vi "Safety_Check.vi"(1 "Adam Loop Count":i32, 2 "Ch Names":string[](array[string]), 3 "Values":dbl[](array[numeric]) format="%.2f") -> (0 "Scan comment":string)   [LabVIEW 2013]
uses:
  ADAM Client/Sub VIs/ADAM Controls/Update_scan_value.ctl
  Anemometry/Anemometry Sub Vis/Globals/Gas_management_global.vi
  ADAM_Global.vi
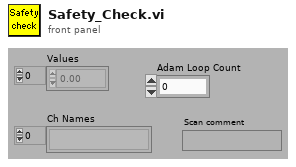
[diagram p1: front panel]
types:
  T1 = cluster{"Channel name":string, "Set value of A to":dbl, "Set value of B to":dbl, "Set value of C to":dbl, "Set value of D to":dbl}
  T2 = typedef "Update_scan_value.ctl" = cluster{"Channel Name":string, "New Value":dbl}
  T3 = enum16{"Append to Global", "Read Global then Clear"}
  T4 = enum16{"On", "Off", "Always On", "Always Off", "Delete"}
  T5 = typedef "LVDateTimeRec.ctl" = cluster{"fractional second":dbl, "second":i32, "minute":i32, "hour":i32, "day of month":i32, "month":i32, "year":i32, "day of week":i32, "day of year":i32, "DST":i32}
  T6 = cluster{"Channel name":string, "Set value of A to":dbl, "Set value of B to":dbl, "Set value of C to":dbl, "Set value of D to":dbl}[]
  T7 = typedef "Ch_description_ADAM.ctl" = cluster{"Ch Name":string, "Type":T8, "Function":T9, "Ch State":T10, "Calibration type":T11, "A":dbl, "B":dbl, "C":dbl, "D":dbl, "Comments":string, "Address":T12, "String":string, "Duty":u16}
  T8 = typedef "Module_type_ADAM.ctl" = string
  T9 = typedef "Function_ADAM.ctl" = enum16{"Analogue Input", "Digital Input", "Event counter", "Event rate", "Analogue Output", "Digital Output", "Relay Output"}
  T10 = typedef "Channel_State.ctl" = enum16{"On", "Off", "Always On", "Always Off"}
  T11 = typedef "Calib_type_ADAM.ctl" = enum16{"Raw", "Bx + A", "Cx^2 + Bx + A", "Dx^3 + Cx^2 + Bx + A", "In Band", "Hi-Tec Q", "Hi-Tec M_dot", "Text"}
  T12 = typedef "Address.ctl" = cluster{"Main":i32, "Ch.":i32, "Sub":i32, "Port Name":string}
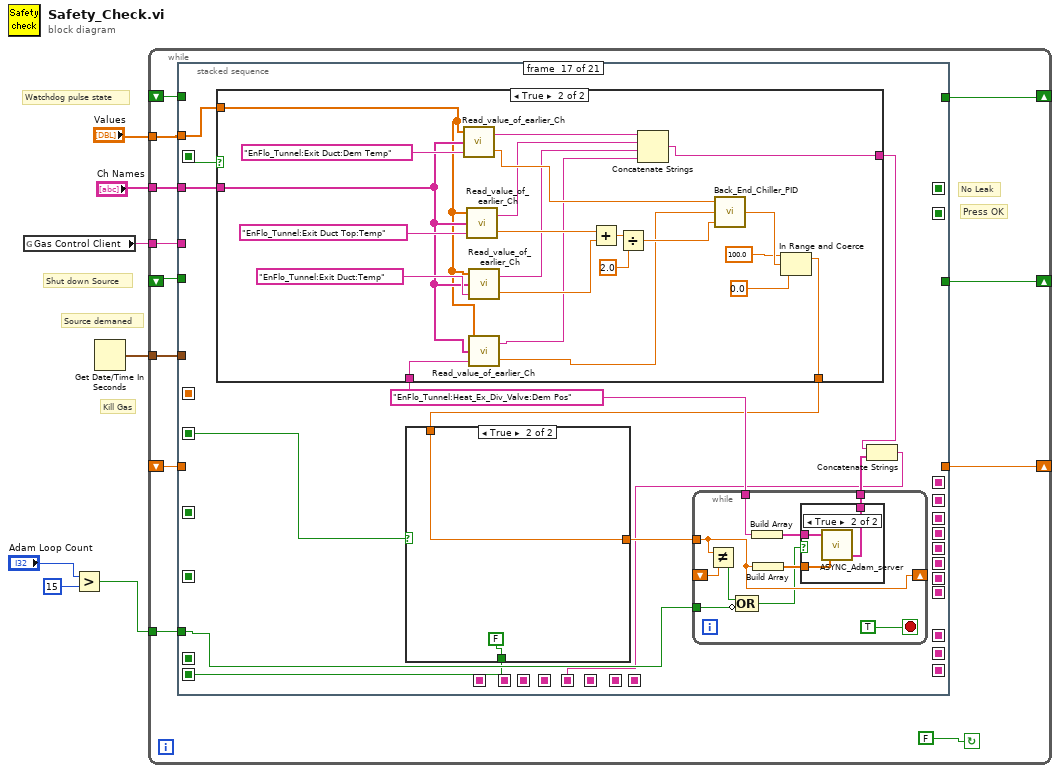
[diagram p0: block diagram]
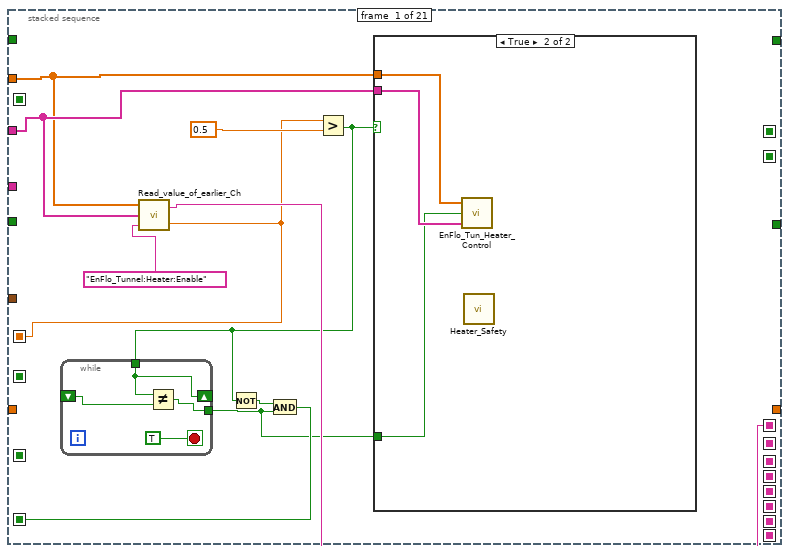
[diagram p2: hidden frame]
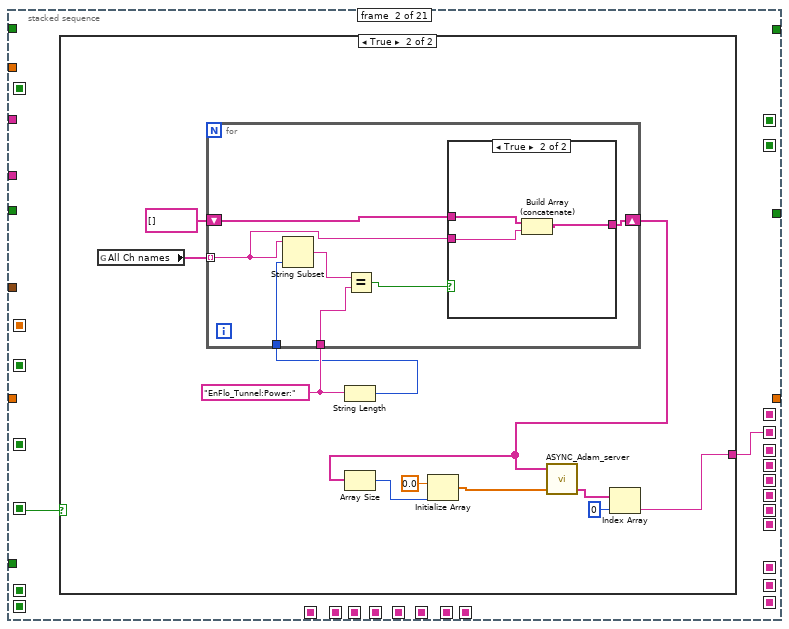
[diagram p4: hidden frame]
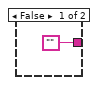
[diagram p5: hidden frame]
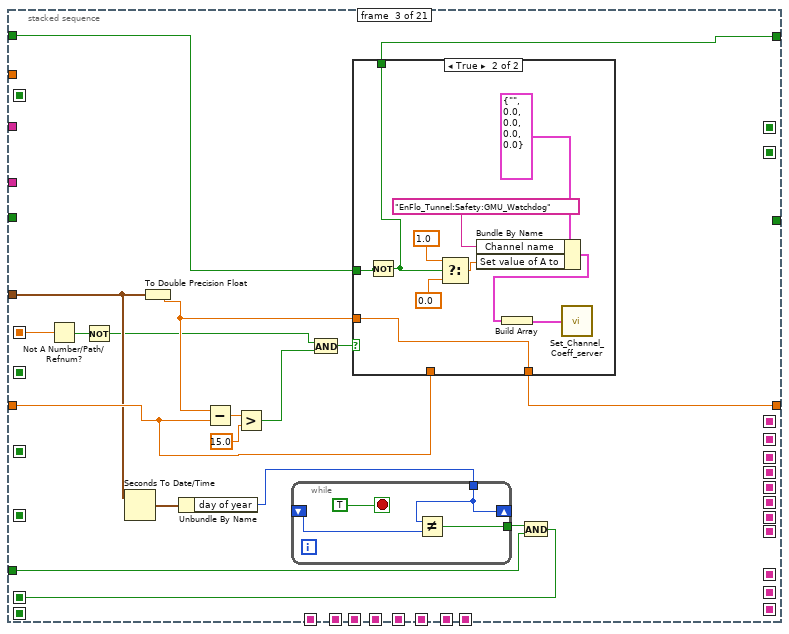
[diagram p7: hidden frame]
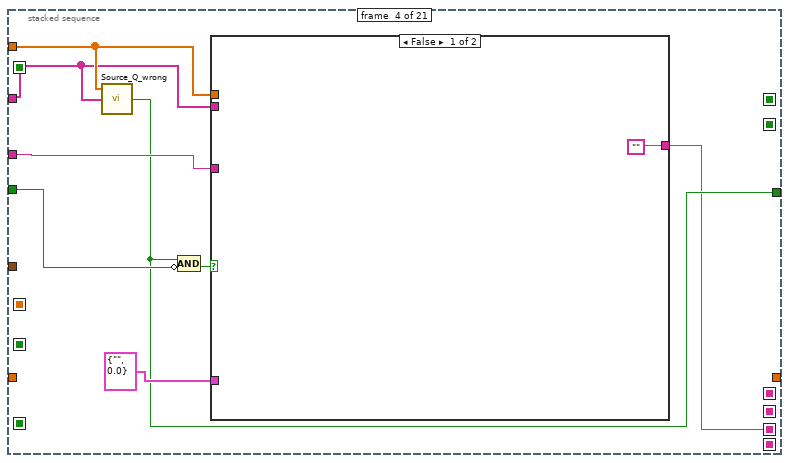
[diagram p9: hidden frame]
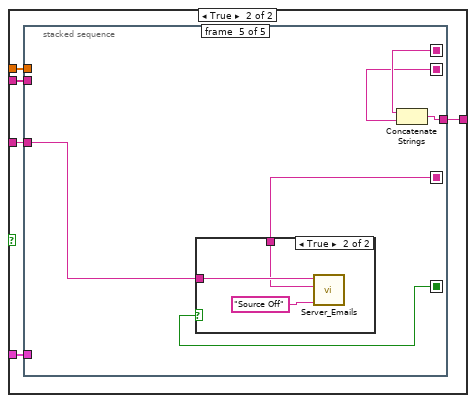
[diagram p10: hidden frame]
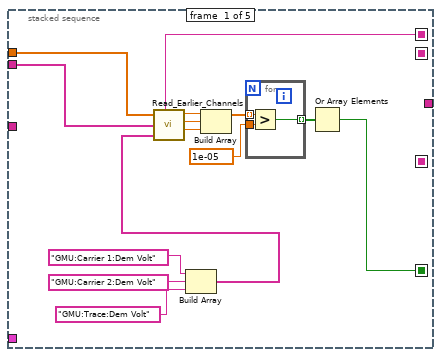
[diagram p11: hidden frame]
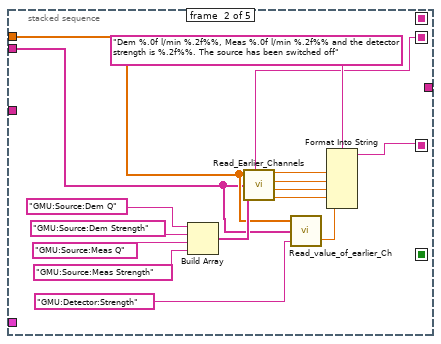
[diagram p12: hidden frame]
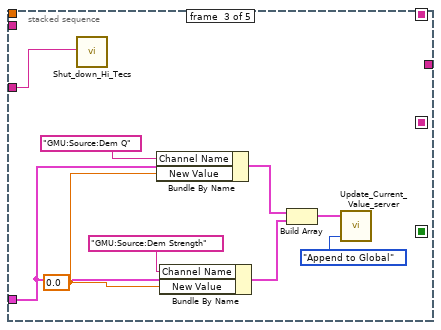
[diagram p13: hidden frame]
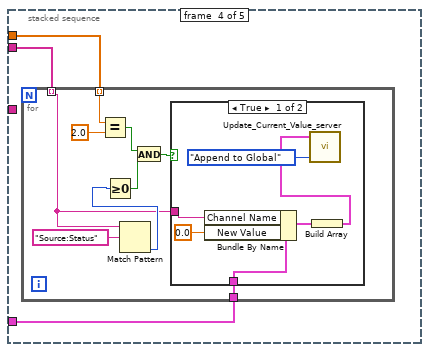
[diagram p14: hidden frame]
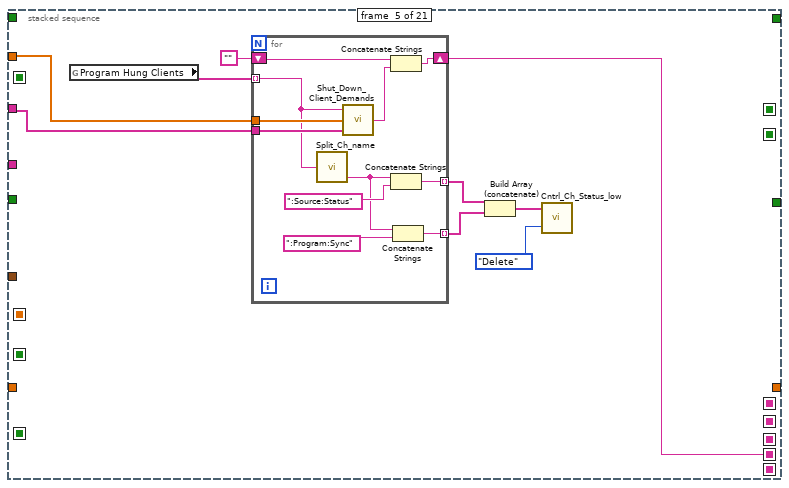
[diagram p17: hidden frame]
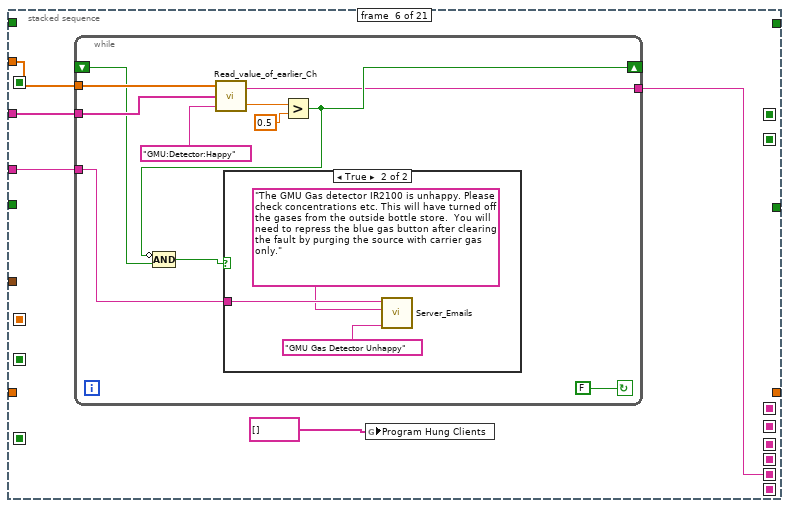
[diagram p18: hidden frame]
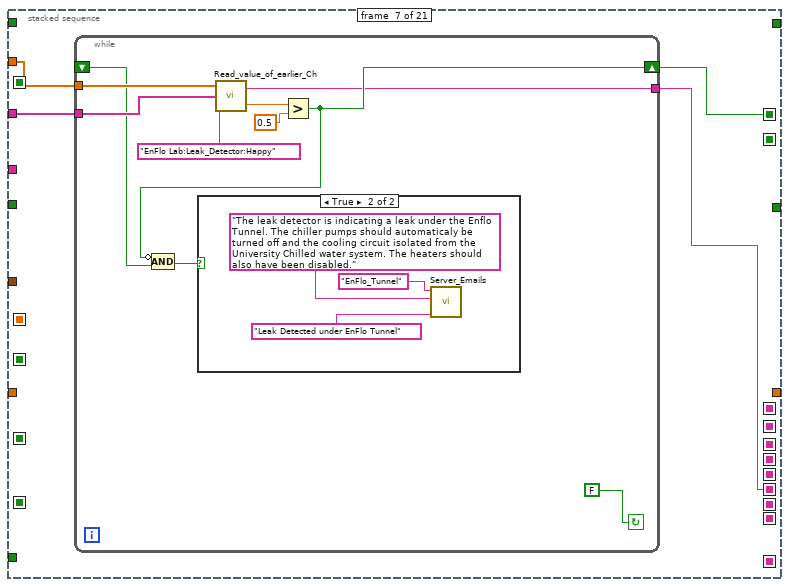
[diagram p20: hidden frame]
diagram:
  # "Shut down Source"
  # "Source demaned"
  # "Watchdog pulse state"
  # "Kill Gas"
  n1 = global read "Gas_management_global.vi" "Gas Control Client"() -> (w5:string)
  n2 = Greater?(x="Adam Loop Count", y=15) -> (0:w2:bool)
  n3 = Get Date/Time In Seconds() -> (seconds since 1Jan1904=w1:timestamp)
  n4 = while {
    shift-left: _ -> [w14]
    shift-right: [w13] -> _
    shift-left: _ -> [w16]
    shift-right: [w15] -> _
    tunnel: w5 -> [w18]
    tunnel: "Ch Names" -> [w19]
    tunnel: "Values" -> [w17]
    shift-right: [w11] -> _
    shift-left: _ -> [w10]
    tunnel: w2 -> [w9]
    tunnel: w1 -> [w8]
    stop <- FALSE continue-if-true
    # "Press OK"
    # "No Leak"
    n5 = stacked-sequence {
      seq-local: [_ _ _ _ _ _ w219 _ _ _ _ _ _ _ _ _ _ _ _ _ _] -> [_ _ _ _ _ _ _ _ _ _ _ _ _ w453 _ _ _ _ _ _ _]
      seq-local: [w22 _ _ _ _ _ _ _ _ _ _ _ _ _ _ _ _ _ _ _ _] -> [_ w38 _ _ _ _ _ _ _ _ _ _ _ _ _ _ _ _ _ _ _]
      seq-local: [_ _ w68 _ _ _ _ _ _ _ _ _ _ _ _ _ _ _ _ _ _] -> [_ _ _ _ _ _ _ _ _ _ _ _ _ _ _ _ _ _ _ _ _]
      seq-local: [_ _ _ _ _ _ _ _ _ _ _ _ _ _ _ w514 _ _ _ _ _] -> [_ _ _ _ _ _ _ _ _ _ _ _ _ _ _ _ w527 _ _ _ _]
      seq-local: [_ _ _ _ _ _ _ _ _ _ _ _ _ _ _ _ w522 _ _ _ _] -> [_ _ _ _ _ _ _ _ _ _ _ _ _ _ _ _ _ _ _ w648 _]
      seq-local: [w25 _ _ _ _ _ _ _ _ _ _ _ _ _ _ _ _ _ _ _ _] -> [_ _ _ _ _ _ _ _ _ _ _ _ _ _ _ _ _ _ _ _ w685]
      seq-local: [_ w37 _ _ _ _ _ _ _ _ _ _ _ _ _ _ _ _ _ _ _] -> [_ _ _ _ _ _ _ _ _ _ _ _ _ _ _ _ _ _ _ _ w684]
      seq-local: [_ _ _ w96 _ _ _ _ _ _ _ _ _ _ _ _ _ _ _ _ _] -> [_ _ _ _ _ _ _ _ _ _ _ _ _ _ _ _ _ _ _ _ w683]
      seq-local: [_ _ _ _ w179 _ _ _ _ _ _ _ _ _ _ _ _ _ _ _ _] -> [_ _ _ _ _ _ _ _ _ _ _ _ _ _ _ _ _ _ _ _ w682]
      seq-local: [_ _ _ _ _ w199 _ _ _ _ _ _ _ _ _ _ _ _ _ _ _] -> [_ _ _ _ _ _ _ _ _ _ _ _ _ _ _ _ _ _ _ _ w681]
      seq-local: [_ _ _ _ _ _ w218 _ _ _ _ _ _ _ _ _ _ _ _ _ _] -> [_ _ _ _ _ _ _ _ _ _ _ _ _ _ _ _ _ _ _ _ w680]
      seq-local: [_ _ _ _ _ _ _ _ _ w330 _ _ _ _ _ _ _ _ _ _ _] -> [_ _ _ _ _ _ _ _ _ _ _ _ _ _ _ _ _ _ _ _ w679]
      seq-local: [_ _ _ _ _ _ _ _ _ _ w362 _ _ _ _ _ _ _ _ _ _] -> [_ _ _ _ _ _ _ _ _ _ _ _ _ _ _ _ _ _ _ _ w670]
      seq-local: [_ _ _ _ _ _ _ _ _ _ _ _ w430 _ _ _ _ _ _ _ _] -> [_ _ _ _ _ _ _ _ _ _ _ _ _ _ _ _ _ _ _ _ w669]
      seq-local: [_ _ _ _ _ _ _ _ _ _ _ _ _ w454 _ _ _ _ _ _ _] -> [_ _ _ _ _ _ _ _ _ _ _ _ _ _ _ _ _ _ _ _ w672]
      seq-local: [_ _ _ _ _ _ _ _ _ _ _ _ _ _ w481 _ _ _ _ _ _] -> [_ _ _ _ _ _ _ _ _ _ _ _ _ _ _ _ _ _ _ _ w673]
      seq-local: [_ _ _ _ _ _ _ _ _ _ _ _ _ _ _ w505 _ _ _ _ _] -> [_ _ _ _ _ _ _ _ _ _ _ _ _ _ _ _ _ _ _ _ w674]
      seq-local: [_ _ _ _ _ _ _ _ _ _ _ _ _ _ _ _ w519 _ _ _ _] -> [_ _ _ _ _ _ _ _ _ _ _ _ _ _ _ _ _ _ _ _ w675]
      seq-local: [_ _ _ _ _ _ _ _ _ _ _ _ _ _ _ _ _ w581 _ _ _] -> [_ _ _ _ _ _ _ _ _ _ _ _ _ _ _ _ _ _ _ _ w676]
      seq-local: [_ _ _ _ _ _ _ _ _ _ _ _ _ _ _ _ _ _ w610 _ _] -> [_ _ _ _ _ _ _ _ _ _ _ _ _ _ _ _ _ _ _ _ w677]
      seq-local: [_ _ _ _ _ _ _ _ _ _ _ _ _ _ _ _ _ _ _ w646 _] -> [_ _ _ _ _ _ _ _ _ _ _ _ _ _ _ _ _ _ _ _ w678]
      seq-local: [w24 _ _ _ _ _ _ _ _ _ _ _ _ _ _ _ _ _ _ _ _] -> [_ _ w66 _ _ _ _ _ _ _ _ _ _ _ _ _ _ _ _ _ _]
      seq-local: [_ _ _ _ _ _ _ _ _ _ _ _ _ _ _ w504 _ _ _ _ _] -> [_ _ _ _ _ _ _ _ _ _ _ _ _ _ _ _ w518 _ _ _ _]
      seq-local: [_ _ _ _ _ _ _ w237 _ _ _ _ _ _ _ _ _ _ _ _ _] -> [_ _ _ _ _ _ _ _ _ _ _ _ _ w452 _ _ _ _ _ _ _]
      seq-local: [_ _ _ _ _ _ _ w236 _ _ _ _ _ _ _ _ _ _ _ _ _] -> [_ _ _ _ _ _ _ _ _ _ _ _ _ _ _ _ _ _ _ _ w668]
      seq-local: [_ _ _ _ _ _ _ w235 _ _ _ _ _ _ _ _ _ _ _ _ _] -> [_ _ _ _ _ _ _ _ w267 _ _ _ _ _ _ _ _ _ _ _ _]
      seq-local: [_ _ _ _ _ _ _ _ w264 _ _ _ _ _ _ _ _ _ _ _ _] -> [_ _ _ _ _ _ _ _ _ _ _ _ _ _ _ _ _ _ _ _ _]
      seq-local: [_ _ _ _ _ _ _ _ _ _ _ w384 _ _ _ _ _ _ _ _ _] -> [_ _ _ _ _ _ _ _ _ _ _ _ _ _ _ _ _ _ _ _ w667]
      tunnel: w19 -> [w27 _ _ w98 w186 w201 w220 w238 w265 w331 w363 w385 w432 w455 w487 w510 w528 w586 w613 _ _]
      tunnel: w18 -> [_ _ _ w103 _ w200 _ _ _ _ _ _ _ _ _ _ _ _ _ _ _]
      tunnel: w17 -> [w26 _ _ w99 w182 w202 w221 w239 w266 w332 w364 w386 w433 w456 w488 w511 w529 w587 w614 _ _]
      tunnel: w16 -> [_ _ w79 _ _ _ _ _ _ _ _ _ _ _ _ _ _ _ _ _ _]
      tunnel: [_ _ w78 _ _ _ _ _ _ _ _ _ _ _ _ _ _ _ _ _ _] -> w15
      tunnel: w14 -> [_ _ _ w102 _ _ _ _ _ _ _ _ _ _ _ _ _ _ _ _ _]
      tunnel: [_ _ _ w97 _ _ _ _ _ _ _ _ _ _ _ _ _ _ _ _ _] -> w13
      tunnel: [_ _ w77 _ _ _ _ _ _ _ _ _ _ _ _ _ _ _ _ _ _] -> w11
      tunnel: w10 -> [_ _ w73 _ _ _ _ _ _ _ _ _ _ _ _ _ _ _ _ _ _]
      tunnel: w9 -> [_ _ w69 _ _ _ _ _ _ _ _ w382 w431 _ _ _ w523 w582 _ w647 _]
      tunnel: w8 -> [_ _ w67 _ _ _ _ _ _ _ _ w383 _ _ _ _ _ _ _ _ _]
      frame #0 {
        n6 = call "Read_value_of_earlier_Ch.vi"("Desired Ch to Read"="EnFlo_Tunnel:Heater:Enable", "Ch names"=w27, "Present scan array"=w26) -> ("Value"=w24:dbl, "Scan comment"=w25:string)  [unwired: 1 in]
        n7 = Greater?(x=w24, y=0.5) -> (0:w23:bool)
        n8 = while {
          shift-right: [w33] -> _
          shift-left: _ -> [w32]
          tunnel: w23 -> [w33]
          tunnel: [w30] -> w20
          stop <- TRUE stop-if-true
          n9 = Not Equal?(x=w33, y=w32) -> (x != y?=w30:bool)
        }
        n10 = Not(x=w23) -> (.not. x?=w21:bool)
        n11 = And(x=w21, y=w20) -> (x .and. y?=w22:bool)
        n12 = case shown="True" w23 {
          tunnel: w26 -> [_ w36]
          tunnel: w27 -> [_ w35]
          tunnel: w20 -> [_ w34]
          frame False {
          }
          frame True {
            n13 = call "EnFlo_Tun_Heater_Control.vi"("Ch Names"=w35, "Heaters Just Enabled"=w34, "Values"=w36) -> ()  [unwired: 1 in]
            n14 = call "Heater_Safety.vi"() -> ()  [unwired: 3 in, 5 out]
          }
        }
      }
      frame #1 {
        n15 = case shown="True" w38 {
          tunnel: ["" w41] -> w37
          frame False {
          }
          frame True {
            w50 = "EnFlo_Tunnel:Power:"
            n16 = global read "ADAM_Global.vi" "All Ch names"() -> (w40:string[])
            n17 = String Length(string=w50) -> (length=w49:i32)
            n18 = for {
              shift-right: [w52] -> w45
              shift-left: string[] [] -> [w53]
              tunnel: w40 -> [w56] mode=indexing
              tunnel: w49 -> [w57]
              tunnel: w50 -> [w54]
              n19 = String Subset(string=w56, length (rest)=w57) -> (substring=w55:string)  [unwired: 1 out]
              n20 = Equal?(x=w55, y=w54) -> (x = y?=w51:bool)
              n21 = case shown="True" w51 {
                tunnel: w56 -> [_ w61]
                tunnel: w53 -> [w58 w59]
                tunnel: [w58 w60] -> w52
                frame False {
                }
                frame True {
                  n22 = Build Array (concatenate)(w59, w61) -> (w60:string[])
                }
              }
            }
            n23 = Array Size(array=w45) -> (size(s)=w46:i32)
            n24 = Initialize Array(0.0 ("element"), w46) -> (w44:dbl[])
            n25 = call "ASYNC_Adam_server.vi"("Values"=w44, "Channel Names"=w45) -> ("Scan Comments"=w43:string[])  [unwired: 1 in, 2 out]
            n26 = Index Array(array=w43, index=0) -> (element=w41:string)
          }
        }
      }
      frame #2 {
        n27 = Not A Number/Path/Refnum?(number/path/refnum=w66) -> (NaN/Path/Refnum?=w65:bool)
        n28 = Not(x=w65) -> (.not. x?=w63:bool)
        n29 = Seconds To Date/Time(time stamp (now)=w67) -> (date time rec=w72:T5)  [unwired: 1 in]
        n30 = To Double Precision Float(number=w67) -> (double precision float=w76:dbl)
        n31 = Unbundle By Name(w72) -> ("day of year"=w71:i32)
        n32 = Subtract(x=w76, y=w73) -> (x-y=w75:dbl)
        n33 = Greater?(x=w75, y=15.0) -> (0:w64:bool)
        n34 = while {
          shift-right: [w83] -> _
          shift-left: _ -> [w82]
          tunnel: w71 -> [w83]
          tunnel: [w81] -> w70
          stop <- TRUE stop-if-true
          n35 = Not Equal?(x=w83, y=w82) -> (x != y?=w81:bool)
        }
        n36 = And(x=w63, y=w64) -> (x .and. y?=w62:bool)
        n37 = case shown="True" w62 {
          tunnel: w79 -> [w84 w88]
          tunnel: [w84 w87] -> w78
          tunnel: [w85 w86] -> w77
          tunnel: w76 -> [_ w86]
          tunnel: w73 -> [w85 _]
          frame False {
          }
          frame True {
            n38 = Not(x=w88) -> (.not. x?=w87:bool)
            n39 = Select(t=1.0 ("Suction"), s=w87, f=0.0 ("Suction")) -> (s? t:f=w91:dbl)
            n40 = Bundle By Name(cluster=T1 {"Channel name"="", "Set value of A to"=0.0, "Set value of B to"=0.0, "Set value of C to"=0.0, "Set value of D to"=0.0}, "Channel name"="EnFlo_Tunnel:Safety:GMU_Watchdog" ("Desired Ch to Read"), "Set value of A to"=w91) -> (w95:T1)
            n41 = Build Array(w95) -> (w90:T6)
            n42 = call "Set_Channel_Coeff_server.vi"("Set Array"=w90) -> ()
          }
        }
        n43 = And(x=w70, y=w69) -> (x .and. y?=w68:bool)
      }
      frame #3 {
        n44 = call "Source_Q_wrong.vi"("Ch Names"=w98, "Values"=w99) -> ("Gas Error?"=w97:bool)  [unwired: 1 out]
        n45 = Compound Arithmetic op=AND(w97, invert w102) -> (w101:bool)
        n46 = case shown="False" w101 {
          tunnel: w103 -> [_ w109]
          tunnel: w99 -> [_ w108]
          tunnel: w98 -> [_ w107]
          tunnel: T2 {"Channel Name"="", "New Value"=0.0} ("Update Scan Value Cluster") -> [_ w106]
          tunnel: ["" w105] -> w96
          frame False {
          }
          frame True {
            n47 = stacked-sequence {
              seq-local: [_ w141 _ _ _] -> [_ _ _ _ w174]
              seq-local: [w111 _ _ _ _] -> [_ _ _ _ w173]
              seq-local: [w110 _ _ _ _] -> [_ _ _ _ w172]
              seq-local: [_ w127 _ _ _] -> [_ _ _ _ w171]
              tunnel: w109 -> [_ _ w144 _ w175]
              tunnel: w108 -> [w121 w131 _ w153 _]
              tunnel: w107 -> [w122 w130 _ w154 _]
              tunnel: w106 -> [_ _ w143 w152 _]
              tunnel: [_ _ _ _ w170] -> w105
              frame #0 {
                n48 = Build Array("GMU:Carrier 1:Dem Volt", "GMU:Carrier 2:Dem Volt", "GMU:Trace:Dem Volt") -> (w123:string[])
                n49 = call "Read_Earlier_Channels.vi"("Present scan array"=w121, "Ch names"=w122, "Desired Channels"=w123) -> ("Scan comments"=w110:string, "Index 0"=w117:dbl, "Index 1"=w116:dbl, "Index 2"=w115:dbl)  [unwired: 2 out]
                n50 = Build Array(w117, w116, w115) -> (w114:dbl[])
                n51 = for {
                  tunnel: w114 -> [w126] mode=indexing
                  tunnel: 1e-05 -> [w125]
                  tunnel: [w124] -> w112 mode=indexing
                  n52 = Greater?(x=w126, y=w125) -> (0:w124:bool)
                }
                n53 = Or Array Elements(Boolean array=w112) -> (logical OR=w111:bool)
              }
              frame #1 {
                n54 = Build Array("GMU:Source:Dem Q", "GMU:Source:Dem Strength", "GMU:Source:Meas Q", "GMU:Source:Meas Strength") -> (w136:string[])
                n55 = call "Read_Earlier_Channels.vi"("Present scan array"=w131, "Ch names"=w130, "Desired Channels"=w136) -> ("Scan comments"=w127:string, "Index 0"=w135:dbl, "Index 1"=w134:dbl, "Index 2"=w133:dbl, "Index 3"=w132:dbl)  [unwired: 1 out]
                n56 = call "Read_value_of_earlier_Ch.vi"("Desired Ch to Read"="GMU:Detector:Strength", "Ch names"=w130, "Present scan array"=w131) -> ("Value"=w128:dbl)  [unwired: 1 in, 1 out]
                n57 = Format Into String(format string="Dem %.0f l/min %.2f%%, Meas %.0f l/min %.2f%% and the detector strength is %.2f%%. The source has been switched off" ("Format String"), w135, w134, w133, w132, w128) -> (resulting string=w141:string)  [unwired: 2 in, 1 out]
              }
              frame #2 {
                w145 = 0.0 ("Bundle Element")
                n58 = call "Shut_down_Hi_Tecs.vi"("Client Name"=w144) -> ()  [unwired: 6 out]
                n59 = Bundle By Name(cluster=w143, "Channel Name"="GMU:Source:Dem Q", "New Value"=w145) -> (w150:T2)
                n60 = Bundle By Name(cluster=w143, "Channel Name"="GMU:Source:Dem Strength", "New Value"=w145) -> (w151:T2)
                n61 = Build Array(w150, w151) -> (w147:T2[])
                n62 = call "Update_Current_Value_server.vi"("Mode"=T3."Append to Global", "Update array in"=w147) -> ()  [unwired: 1 in, 1 out]
              }
              frame #3 {
                n63 = for {
                  tunnel: w154 -> [w155] mode=indexing
                  tunnel: w153 -> [w161] mode=indexing
                  tunnel: w152 -> [w156]
                  n64 = Equal?(x=w161, y=2.0) -> (x = y?=w158:bool)
                  n65 = Match Pattern(string=w155, regular expression="Source:Status") -> (offset past match=w162:i32)  [unwired: 4 out]
                  n66 = Greater Or Equal To 0?(x=w162) -> (x >= 0?=w159:bool)
                  n67 = And(x=w158, y=w159) -> (x .and. y?=w157:bool)
                  n68 = case shown="True" w157 {
                    tunnel: w156 -> [w169 _]
                    tunnel: w155 -> [w168 _]
                    frame True {
                      n69 = Bundle By Name(cluster=w169, "Channel Name"=w168, "New Value"=0.0) -> (w166:T2)
                      n70 = Build Array(w166) -> (w165:T2[])
                      n71 = call "Update_Current_Value_server.vi"("Mode"=T3."Append to Global", "Update array in"=w165) -> ()  [unwired: 1 in, 1 out]
                    }
                    frame False {
                    }
                  }
                }
              }
              frame #4 {
                n72 = case shown="True" w173 {
                  tunnel: w175 -> [_ w178]
                  tunnel: w174 -> [_ w177]
                  frame False {
                  }
                  frame True {
                    n73 = call "Server_Emails.vi"("Client Name Contains"=w178, "Message"=w177, "Subject"="Source Off") -> ()  [unwired: 2 in, 3 out]
                  }
                }
                n74 = Concatenate Strings(w172, w171) -> (w170:string)
              }
            }
          }
        }
      }
      frame #4 {
        n75 = global read "ADAM_Global.vi" "Program Hung Clients"() -> (w187:string[])
        n76 = for {
          tunnel: w187 -> [w196] mode=indexing
          tunnel: w182 -> [w198]
          tunnel: w186 -> [w197]
          tunnel: [w194] -> w185 mode=indexing
          tunnel: [w191] -> w184 mode=indexing
          shift-right: [w189] -> w179
          shift-left: "" -> [w190]
          n77 = call "Split_Ch_name.vi"("Ch name"=w196) -> ("Low level"=w193:string)  [unwired: 2 out]
          n78 = call "Shut_Down_Client_Demands.vi"("Ch Names"=w197, "Values"=w198, "Client Name"=w196) -> ("Comments"=w188:string)
          n79 = Concatenate Strings(w190, w188) -> (w189:string)
          n80 = Concatenate Strings(w193, ":Source:Status") -> (w194:string)
          n81 = Concatenate Strings(w193, ":Program:Sync") -> (w191:string)
        }
        n82 = Build Array (concatenate)(w185, w184) -> (w183:string[])
        n83 = call "Cntrl_Ch_Status_low.vi"("Mode"=T4."Delete", "Channel names"=w183) -> ()  [unwired: 1 out]
      }
      frame #5 {
        n84 = while {
          tunnel: w202 -> [w214]
          tunnel: w201 -> [w213]
          shift-right: [w208] -> _
          shift-left: _ -> [w209]
          tunnel: w200 -> [w206]
          tunnel: [w204] -> w199
          stop <- FALSE continue-if-true
          n85 = call "Read_value_of_earlier_Ch.vi"("Desired Ch to Read"="GMU:Detector:Happy", "Ch names"=w213, "Present scan array"=w214) -> ("Value"=w211:dbl, "Scan comment"=w204:string)  [unwired: 1 in]
          n86 = Greater?(x=w211, y=0.5) -> (0:w208:bool)
          n87 = Compound Arithmetic op=AND(invert w208, w209) -> (w207:bool)
          n88 = case shown="True" w207 {
            tunnel: w206 -> [_ w216]
            frame False {
            }
            frame True {
              n89 = call "Server_Emails.vi"("Client Name Contains"=w216, "Message"="The GMU Gas detector IR2100 is unhappy. Please check concentrations etc. This will have turned off the gases from the outside bottle store.  You will need to repress the blue gas button after clearing the fault by purging the source with carrier gas only.", "Subject"="GMU Gas Detector Unhappy") -> ()  [unwired: 2 in, 3 out]
            }
          }
        }
        n90 = global write "ADAM_Global.vi" "Program Hung Clients"(string[] [] ("Program Hung Clients")) -> ()
      }
      frame #6 {
        n91 = while {
          tunnel: w221 -> [w231]
          tunnel: w220 -> [w230]
          shift-right: [w225] -> w219
          shift-left: _ -> [w226]
          tunnel: [w222] -> w218
          stop <- FALSE continue-if-true
          n92 = call "Read_value_of_earlier_Ch.vi"("Desired Ch to Read"="EnFlo Lab:Leak_Detector:Happy", "Ch names"=w230, "Present scan array"=w231) -> ("Value"=w228:dbl, "Scan comment"=w222:string)  [unwired: 1 in]
          n93 = Greater?(x=w228, y=0.5) -> (0:w225:bool)
          n94 = Compound Arithmetic op=AND(invert w225, w226) -> (w224:bool)
          n95 = case shown="True" w224 {
            frame False {
            }
            frame True {
              n96 = call "Server_Emails.vi"("Client Name Contains"="EnFlo_Tunnel", "Message"="The leak detector is indicating a leak under the Enflo Tunnel. The chiller pumps should automaticaly be turned off and the cooling circuit isolated from the  University Chilled water system. The heaters should also have been disabled.", "Subject"="Leak Detected under EnFlo Tunnel") -> ()  [unwired: 2 in, 3 out]
            }
          }
        }
      }
      frame #7 {
        n97 = while {
          tunnel: w239 -> [w245]
          tunnel: w238 -> [w244]
          shift-right: [w256] -> w237
          shift-left: _ -> [w257]
          tunnel: [w248] -> w236
          tunnel: [w240] -> w235
          stop <- FALSE continue-if-true
          n98 = call "Read_value_of_earlier_Ch.vi"("Desired Ch to Read"="EnFlo_Tunnel:Chiller_Pump:Enable", "Ch names"=w244, "Present scan array"=w245) -> ("Value"=w251:dbl, "Scan comment"=w249:string)  [unwired: 1 in]
          n99 = call "Read_value_of_earlier_Ch.vi"("Desired Ch to Read"="EnFlo_Tunnel:Chilled Water:Pressure_OK", "Ch names"=w244, "Present scan array"=w245) -> ("Value"=w259:dbl, "Scan comment"=w250:string)  [unwired: 1 in]
          n100 = call "Read_value_of_earlier_Ch.vi"("Desired Ch to Read"="EnFlo_Tunnel:Chiller_Pump:Running", "Ch names"=w244, "Present scan array"=w245) -> ("Value"=w242:dbl, "Scan comment"=w241:string)  [unwired: 1 in]
          n101 = Greater?(x=w259, y=0.5) -> (0:w256:bool)
          n102 = Greater?(x=w251, y=0.5) -> (0:w247:bool)
          n103 = Compound Arithmetic op=AND(invert w256, w257, w247) -> (w255:bool)
          n104 = case shown="True" w255 {
            frame False {
            }
            frame True {
              n105 = call "Server_Emails.vi"("Client Name Contains"="EnFlo_Tunnel", "Message"="The pressure in the chilled water  for the Enflo Tunnel has tripped the system. The chiller pumps should automaticaly be turned off and the cooling circuit isolated from the  University Chilled water system. The heaters should also have been disabled.", "Subject"="EnFlo Chilled Water Overpressure Trip") -> ()  [unwired: 2 in, 3 out]
            }
          }
          n106 = Greater?(x=w242, y=0.5) -> (0:w240:bool)
          n107 = Concatenate Strings(w249, w250, w241) -> (w248:string)
        }
      }
      frame #8 {
        n108 = case shown="True" w267 {
          tunnel: w266 -> [_ w294]
          tunnel: w265 -> [_ w293]
          tunnel: ["" w273] -> w264
          frame False {
          }
          frame True {
            w278 = "EnFlo_Tunnel:Chilled Water:Motor_Dem_Voltage"
            # "EnFlo_Tunnel:Chiller_Pump:Running"
            n109 = call "Read_value_of_earlier_Ch.vi"("Desired Ch to Read"="EnFlo_Tunnel:Chilled Water:Pressure_supply (Bar)", "Ch names"=w293, "Present scan array"=w294) -> ("Value"=w270:dbl, "Scan comment"=w277:string)  [unwired: 1 in]
            n110 = call "Read_value_of_earlier_Ch.vi"("Desired Ch to Read"="EnFlo_Tunnel:Chilled Water:Pressure_return (Bar)", "Ch names"=w293, "Present scan array"=w294) -> ("Value"=w289:dbl, "Scan comment"=w276:string)  [unwired: 1 in]
            n111 = call "Read_value_of_earlier_Ch.vi"("Desired Ch to Read"="EnFlo_Tunnel:Chilled Water:Desired_Delta_P", "Ch names"=w293, "Present scan array"=w294) -> ("Value"=w287:dbl, "Scan comment"=w275:string)  [unwired: 1 in]
            n112 = call "Read_value_of_earlier_Ch.vi"("Desired Ch to Read"=w278, "Ch names"=w293, "Present scan array"=w294) -> ("Value"=w282:dbl, "Scan comment"=w274:string)  [unwired: 1 in]
            n113 = Subtract(x=w270, y=w289) -> (x-y=w288:dbl)
            n114 = Subtract(x=w288, y=w287) -> (x-y=w281:dbl)
            n115 = Concatenate Strings(w277, w276, w275, w274) -> (w273:string)
            n116 = In Range and Coerce(upper limit=0.1 ("lower limit"), x=w281, lower limit=-0.1) -> (In Range?=w272:bool)  [unwired: 1 out]
            n117 = Less?(x=w270, y=3.85) -> (x < y?=w269:bool)
            n118 = Less?(x=w270, y=4.0) -> (x < y?=w283:bool)
            n119 = case shown="True" w283 {
              tunnel: w282 -> [w305 w309]
              tunnel: w272 -> [_ w311]
              tunnel: w281 -> [_ w310]
              tunnel: [TRUE w308] -> w280
              tunnel: [w302 w307] -> w279
              tunnel: w269 -> [_ w306]
              frame False {
                n120 = Subtract(x=w305, y=0.2) -> (x-y=w302:dbl)
              }
              frame True {
                n121 = case shown="False" w311 {
                  tunnel: w310 -> [w317 _]
                  tunnel: w309 -> [w316 w328]
                  tunnel: [TRUE FALSE] -> w308
                  tunnel: [w314 w328] -> w307
                  tunnel: w306 -> [w312 _]
                  frame False {
                    n122 = Greater Than 0?(x=w317) -> (x > 0?=w315:bool)
                    n123 = case shown="False" w315 {
                      tunnel: w316 -> [w319 w323]
                      tunnel: [w318 w322] -> w314
                      tunnel: w312 -> [_ w321]
                      frame True {
                        n124 = Subtract(x=w319, y=0.1) -> (x-y=w318:dbl)
                      }
                      frame False {
                        n125 = case shown="False" w321 {
                          tunnel: w323 -> [w324 w326]
                          tunnel: [w324 w325] -> w322
                          frame False {
                          }
                          frame True {
                            n126 = Add(x=w326, y=0.1) -> (x+y=w325:dbl)
                          }
                        }
                      }
                    }
                  }
                  frame True {
                  }
                }
              }
            }
            n127 = case shown="True" w280 {
              tunnel: w279 -> [_ w296]
              tunnel: w278 -> [_ w299]
              frame False {
              }
              frame True {
                n128 = In Range and Coerce(upper limit=10.0, x=w296, lower limit=0.0) -> (coerced(x)=w295:dbl)  [unwired: 1 out]
                n129 = Build Array(w299) -> (w300:string[])
                n130 = Build Array(w295) -> (w301:dbl[])
                n131 = call "ASYNC_Adam_server.vi"("Values"=w301, "Channel Names"=w300) -> ()  [unwired: 1 in, 3 out]
              }
            }
          }
        }
      }
      frame #9 {
        n132 = while {
          tunnel: w332 -> [w348]
          tunnel: w331 -> [w347]
          shift-right: [w341] -> _
          shift-left: _ -> [w337]
          tunnel: [w333] -> w330
          stop <- FALSE continue-if-true
          w339 = 60.0 ("y")
          n133 = Decrement(x=w339) -> (x-1=w340:dbl)
          n134 = Select(t=w340, s=w337, f=w339) -> (s? t:f=w338:dbl)
          n135 = call "Read_value_of_earlier_Ch.vi"("Desired Ch to Read"="EnFlo_Tunnel:Chilled Water:Motor1 Temp", "Ch names"=w347, "Present scan array"=w348) -> ("Value"=w355:dbl, "Scan comment"=w335:string)  [unwired: 1 in]
          n136 = call "Read_value_of_earlier_Ch.vi"("Desired Ch to Read"="EnFlo_Tunnel:Chilled Water:Motor2 Temp", "Ch names"=w347, "Present scan array"=w348) -> ("Value"=w352:dbl, "Scan comment"=w334:string)  [unwired: 1 in]
          n137 = Greater?(x=w355, y=w338) -> (0:w349:bool)
          n138 = Greater?(x=w352, y=w338) -> (0:w350:bool)
          n139 = Or(x=w349, y=w350) -> (x .or. y?=w343:bool)
          n140 = call "Read_value_of_earlier_Ch.vi"("Desired Ch to Read"="EnFlo_Tunnel:Chiller_Pump:Enable", "Ch names"=w347, "Present scan array"=w348) -> ("Value"=w345:dbl, "Scan comment"=w336:string)  [unwired: 1 in]
          n141 = Greater?(x=w345, y=0.5) -> (0:w342:bool)
          n142 = And(x=w342, y=w343) -> (x .and. y?=w341:bool)
          n143 = Compound Arithmetic op=AND(w341, invert w337) -> (w354:bool)
          n144 = case shown="True" w354 {
            tunnel: w339 -> [_ w358]
            frame False {
            }
            frame True {
              n145 = Format Into String(format string="The Chilled Water Motor Temp is greater than %.0f deg C." ("Message"), w358) -> (resulting string=w357:string)  [unwired: 2 in, 1 out]
              n146 = call "Server_Emails.vi"("Client Name Contains"="EnFlo_Tunnel", "Message"=w357, "Subject"="Chilled Water Motor Temp") -> ()  [unwired: 2 in, 3 out]
            }
          }
          n147 = Concatenate Strings(w336, w335, w334) -> (w333:string)
        }
      }
      frame #10 {
        n148 = while {
          tunnel: w364 -> [w378]
          tunnel: w363 -> [w377]
          shift-right: [w366] -> _
          shift-left: _ -> [w372]
          shift-left: _ -> [w371]
          shift-left: _ -> [w370]
          tunnel: [w365] -> w362
          stop <- FALSE continue-if-true
          n149 = call "Read_value_of_earlier_Ch.vi"("Desired Ch to Read"="FFID:System:Enable", "Ch names"=w377, "Present scan array"=w378) -> ("Value"=w373:dbl, "Scan comment"=w365:string)  [unwired: 1 in]
          n150 = Greater?(x=w373, y=0.5) -> (0:w366:bool)
          n151 = Compound Arithmetic op=AND(w366, w372, invert w371, invert w370) -> (w368:bool)
          n152 = Compound Arithmetic op=AND(invert w366, invert w372, w371, w370) -> (w369:bool)
          n153 = Or(x=w368, y=w369) -> (x .or. y?=w367:bool)
          n154 = case shown="False" w367 {
            tunnel: w373 -> [_ w379]
            tunnel: w366 -> [_ _]
            frame False {
            }
            frame True {
              n155 = Build Array(w379) -> (w381:dbl[])
              n156 = call "ASYNC_Adam_server.vi"("Values"=w381, "Channel Names"=string[] ["GMU:Gas:Enable"]) -> ()  [unwired: 1 in, 3 out]
            }
          }
        }
      }
      frame #11 {
        n157 = while {
          tunnel: w386 -> [w398]
          tunnel: w385 -> [w397]
          shift-right: [w388] -> _
          shift-left: _ -> [w393]
          tunnel: [w392] -> w384
          tunnel: w383 -> [w390]
          tunnel: w382 -> [w387]
          stop <- FALSE continue-if-true
          w389 = "EnFlo_Tunnel:Motor:Enable" ("Desired Ch to Read")
          # "Re Zero EnFlo Tunnel static pressure when turning tunnel on"
          n158 = call "Read_value_of_earlier_Ch.vi"("Desired Ch to Read"=w389, "Ch names"=w397, "Present scan array"=w398) -> ("Value"=w394:dbl, "Scan comment"=w392:string)  [unwired: 1 in]
          n159 = Greater?(x=w394, y=0.5) -> (0:w388:bool)
          n160 = Compound Arithmetic op=AND(w388, invert w393, w387) -> (w391:bool)
          n161 = case shown="False" w391 {
            tunnel: w390 -> [_ w424]
            tunnel: w389 -> [_ w422]
            frame False {
            }
            frame True {
              w421 = "EnFlo_Tunnel:Pressure:Static"
              n162 = To Double Precision Float(number=w424) -> (double precision float=w407:dbl)
              n163 = Build Array(w421) -> (w420:string[])
              n164 = Build Array(w422, w421) -> (w425:string[])
              n165 = Subtract(x=w407, y=15.0) -> (x-y=w405:dbl)
              n166 = call "Get_Current_Scan_server.vi"("Desired Channels"=w420) -> ("Ch Description Array"=w419:T7[])  [unwired: 2 out]
              n167 = Subtract(x=w407, y=3600.0) -> (x-y=w423:dbl)
              n168 = call "Get_ADAM_averages_server.vi"("No of averages"=600, "End time"=w405, "Start time"=w423, "Clients time"=w407, "ADAM Ch Names"=w425) -> ("DBL values"=w409:dbl[][])  [unwired: 1 in, 4 out]
              n169 = Index Array(array=w419) -> (element=w417:T7)  [unwired: 1 in]
              n170 = Unbundle By Name(w417) -> ("A"=w418:dbl)
              n171 = Index Array(array=w409, index (col)=1 ("disabled index (col)")) -> (element=w404:dbl[])  [unwired: 1 in]
              n172 = Index Array(array=w409, index (col)=2 ("disabled index (col)")) -> (element=w403:dbl[])  [unwired: 1 in]
              n173 = Reverse 1D Array(array=w403) -> (reversed array=w399:dbl[])
              n174 = Reverse 1D Array(array=w404) -> (reversed array=w402:dbl[])
              n175 = for {
                tunnel: w402 -> [w427] mode=indexing
                tunnel: [w426] -> w401 mode=indexing
                tunnel: w399 -> [w426] mode=indexing
                stop <- w428 continue-if-true
                n176 = Less?(x=w427, y=0.01) -> (x < y?=w428:bool)
              }
              n177 = call "Mean_fr_NaN_data.vi"("Data"=w401) -> ("Mean value"=w400:dbl)  [unwired: 1 out]
              n178 = Subtract(x=w418, y=w400) -> (x-y=w416:dbl)
              n179 = Bundle By Name(cluster=w417, "A"=w416) -> (w415:T7)
              n180 = Build Array(w415) -> (w414:T7[])
              n181 = call "Update_Ch_Discription_server.vi"("Mode"=T3."Append to Global", "Channels to update In"=w414) -> ()  [unwired: 1 in, 1 out]
            }
          }
        }
      }
      frame #12 {
        # "Resetting A Tunnel speed to zero if the drive in turned off\nso that the belts do not slip when the tunnel is turned on again."
        n182 = while {
          tunnel: w433 -> [w446]
          tunnel: w432 -> [w445]
          shift-right: [w437] -> _
          shift-left: _ -> [w440]
          shift-left: _ -> [w439]
          shift-left: _ -> [w438]
          tunnel: w431 -> [w436]
          tunnel: [w434] -> w430
          stop <- FALSE continue-if-true
          n183 = call "Read_value_of_earlier_Ch.vi"("Desired Ch to Read"="A_Tunnel:Motor:Enable", "Ch names"=w445, "Present scan array"=w446) -> ("Value"=w441:dbl, "Scan comment"=w434:string)  [unwired: 1 in]
          n184 = Less?(x=w441, y=0.5) -> (x < y?=w437:bool)
          n185 = Compound Arithmetic op=AND(w437, w440, invert w439, invert w438, w436) -> (w435:bool)
          n186 = case shown="True" w435 {
            tunnel: w437 -> [_ _]
            frame False {
            }
            frame True {
              w449 = string[] ["A_Tunnel:Speed:Dem Velocity", "A_Tunnel:Speed:Dem Voltage"] ("Channel Names")
              n187 = Array Size(array=w449) -> (size(s)=w450:i32)
              n188 = Initialize Array(0.0 ("element"), w450) -> (w448:dbl[])
              n189 = call "ASYNC_Adam_server.vi"("Values"=w448, "Channel Names"=w449) -> ()  [unwired: 1 in, 3 out]
            }
          }
        }
      }
      frame #13 {
        n190 = And(x=w452, y=w453) -> (x .and. y?=w451:bool)
        n191 = case shown="False" w451 {
          tunnel: w456 -> [w461 _]
          tunnel: w455 -> [w460 _]
          tunnel: [w457 ""] -> w454
          frame False {
            n192 = for {
              tunnel: w461 -> [w471]
              tunnel: w460 -> [w470]
              tunnel: string[] ["EnFlo_Tunnel:Heater:Enable", "EnFlo_Tunnel:Chiller_Pump:Enable", "EnFlo_Tunnel:Tap_Water:Enable"] ("Ch Names") -> [w466] mode=indexing
              shift-right: [w464] -> w457
              shift-left: "" -> [w465]
              n193 = call "Read_value_of_earlier_Ch.vi"("Desired Ch to Read"=w466, "Ch names"=w470, "Present scan array"=w471) -> ("Value"=w468:dbl, "Scan comment"=w463:string)  [unwired: 1 in]
              n194 = Greater?(x=w468, y=0.5) -> (0:w467:bool)
              n195 = case shown="True" w467 {
                tunnel: w466 -> [_ w476]
                tunnel: ["" w473] -> w462
                frame False {
                }
                frame True {
                  n196 = Build Array(w476) -> (w479:string[])
                  n197 = Build Array(0.0) -> (w478:dbl[])
                  n198 = call "ASYNC_Adam_server.vi"("Values"=w478, "Channel Names"=w479) -> ("Scan Comments"=w474:string[])  [unwired: 1 in, 2 out]
                  n199 = Index Array(array=w474, index=0) -> (element=w473:string)
                }
              }
              n200 = Concatenate Strings(w465, w463, w462) -> (w464:string)
            }
          }
          frame True {
          }
        }
      }
      frame #14 {
        w489 = "EnFlo_Tunnel:Heater:Enable" ("Ch Name")
        n201 = call "Read_value_of_earlier_Ch.vi"("Desired Ch to Read"=w489, "Ch names"=w487, "Present scan array"=w488) -> ("Value"=w494:dbl, "Scan comment"=w483:string)  [unwired: 1 in]
        n202 = call "Read_value_of_earlier_Ch.vi"("Desired Ch to Read"="EnFlo_Tunnel:Reference:Velocity", "Ch names"=w487, "Present scan array"=w488) -> ("Value"=w491:dbl, "Scan comment"=w482:string)  [unwired: 1 in]
        n203 = Greater?(x=w494, y=0.5) -> (0:w486:bool)
        n204 = Less?(x=w491, y=0.25) -> (x < y?=w490:bool)
        n205 = And(x=w486, y=w490) -> (x .and. y?=w485:bool)
        n206 = case shown="True" w485 {
          tunnel: w489 -> [_ w500]
          tunnel: ["" w497] -> w484
          frame False {
          }
          frame True {
            n207 = Build Array(w500) -> (w503:string[])
            n208 = Build Array(0.0) -> (w502:dbl[])
            n209 = call "ASYNC_Adam_server.vi"("Values"=w502, "Channel Names"=w503) -> ("Scan Comments"=w498:string[])  [unwired: 1 in, 2 out]
            n210 = Index Array(array=w498, index=0) -> (element=w497:string)
          }
        }
        n211 = Concatenate Strings(w483, w482, w484) -> (w481:string)
      }
      frame #15 {
        n212 = call "Read_value_of_earlier_Ch.vi"("Desired Ch to Read"="EnFlo_Tunnel:Chiller_Pump:Running", "Ch names"=w510, "Present scan array"=w511) -> ("Value"=w512:dbl, "Scan comment"=w507:string)  [unwired: 1 in]
        n213 = call "Read_value_of_earlier_Ch.vi"("Desired Ch to Read"="EnFlo_Tunnel:Reference:Velocity", "Ch names"=w510, "Present scan array"=w511) -> ("Value"=w508:dbl, "Scan comment"=w506:string)  [unwired: 1 in]
        n214 = Greater?(x=w508, y=0.4) -> (0:w516:bool)
        n215 = Greater?(x=w512, y=0.5) -> (0:w504:bool)
        n216 = Compound Arithmetic op=AND(w504, w516) -> (w514:bool)
        n217 = Concatenate Strings(w507, w506) -> (w505:string)
      }
      frame #16 {
        w526 = "EnFlo_Tunnel:Heat_Ex_Div_Valve:Dem Pos"
        n218 = case shown="True" w527 {
          tunnel: w529 -> [_ w564]
          tunnel: w528 -> [_ w565]
          tunnel: w526 -> [_ w568]
          tunnel: [0.0 ("upper limit") w574] -> w524
          tunnel: ["" w559] -> w521
          frame False {
          }
          frame True {
            n219 = call "Read_value_of_earlier_Ch.vi"("Desired Ch to Read"="EnFlo_Tunnel:Exit Duct:Dem Temp", "Ch names"=w565, "Present scan array"=w564) -> ("Value"=w573:dbl, "Scan comment"=w563:string)  [unwired: 1 in]
            n220 = call "Read_value_of_earlier_Ch.vi"("Desired Ch to Read"="EnFlo_Tunnel:Exit Duct Top:Temp", "Ch names"=w565, "Present scan array"=w564) -> ("Value"=w569:dbl, "Scan comment"=w562:string)  [unwired: 1 in]
            n221 = call "Read_value_of_earlier_Ch.vi"("Desired Ch to Read"="EnFlo_Tunnel:Exit Duct:Temp", "Ch names"=w565, "Present scan array"=w564) -> ("Value"=w570:dbl, "Scan comment"=w561:string)  [unwired: 1 in]
            n222 = call "Read_value_of_earlier_Ch.vi"("Desired Ch to Read"=w568, "Ch names"=w565, "Present scan array"=w564) -> ("Value"=w571:dbl, "Scan comment"=w560:string)  [unwired: 1 in]
            n223 = Add(x=w569, y=w570) -> (x+y=w578:dbl)
            n224 = Divide(x=w578, y=2.0) -> (x/y=w580:dbl)
            n225 = Concatenate Strings(w563, w562, w561, w560) -> (w559:string)
            n226 = call "Back_End_Chiller_PID.vi"("Present Value"=w580, "Previous Control Sum"=w571, "Setpoint"=w573) -> ("Dem Output"=w577:dbl)
            n227 = In Range and Coerce(upper limit=100.0, x=w577, lower limit=0.0) -> (coerced(x)=w574:dbl)  [unwired: 1 out]
          }
        }
        n228 = case shown="True" w518 {
          tunnel: [w531 w542] -> w525
          tunnel: w524 -> [_ w542]
          tunnel: [w530 FALSE] -> w522
          frame False {
            # "Exercise valve once a week"
            n229 = Seconds To Date/Time() -> (date time rec=w532:T5)  [unwired: 2 out]
            n230 = Unbundle By Name(w532) -> ("day of week"=w537:i32, "hour"=w535:i32)
            n231 = Less?(x=w535, y=3) -> (x < y?=w540:bool)
            n232 = Equal?(x=7, y=w537) -> (x = y?=w539:bool)
            n233 = And(x=w539, y=w540) -> (x .and. y?=w530:bool)
            n234 = Select(t=100.0, s=w530, f=0.0) -> (s? t:f=w531:dbl)
          }
          frame True {
          }
        }
        n235 = while {
          shift-right: [w548] -> _
          shift-left: _ -> [w549]
          tunnel: w525 -> [w548]
          tunnel: w526 -> [w550]
          tunnel: w523 -> [w545]
          tunnel: [w543] -> w520
          stop <- TRUE stop-if-true
          n236 = Not Equal?(x=w548, y=w549) -> (x != y?=w546:bool)
          n237 = Compound Arithmetic op=OR(w546, invert w545) -> (w544:bool)
          n238 = Build Array(w550) -> (w551:string[])
          n239 = Build Array(w548) -> (w552:dbl[])
          n240 = case shown="True" w544 {
            tunnel: w552 -> [_ w556]
            tunnel: w551 -> [_ w555]
            tunnel: [string[] [] ("Scan Comments") w554] -> w543
            frame False {
            }
            frame True {
              n241 = call "ASYNC_Adam_server.vi"("Values"=w556, "Channel Names"=w555) -> ("Scan Comments"=w554:string[])  [unwired: 1 in, 2 out]
            }
          }
        }
        n242 = Concatenate Strings(w521, w520) -> (w519:string)
      }
      frame #17 {
        n243 = Search 1D Array(1D array=w586, element="Status:of:EnFlo_Tunnel") -> (index of element=w589:i32)  [unwired: 1 out]
        n244 = Index Array(array=w587, index=w589) -> (element=w585:dbl)
        n245 = case shown="0, Default" w585 {
          tunnel: [0.0 1.0 1.0 1.0] -> w584
          frame 0, Default {
          }
          frame 1 {
          }
          frame 2 {
          }
          frame 3 {
          }
        }
        n246 = while {
          shift-right: [w599] -> _
          shift-left: _ -> [w600]
          tunnel: w584 -> [w599]
          tunnel: "EnFlo_Tunnel:Warning_Cone:Enable" -> [w601]
          tunnel: w582 -> [w596]
          tunnel: [w594] -> w581
          stop <- TRUE stop-if-true
          n247 = Not Equal?(x=w599, y=w600) -> (x != y?=w597:bool)
          n248 = Build Array(w601) -> (w602:string[])
          n249 = Build Array(w599) -> (w603:dbl[])
          n250 = Compound Arithmetic op=OR(w597, invert w596) -> (w595:bool)
          n251 = case shown="True" w595 {
            tunnel: w603 -> [_ w609]
            tunnel: w602 -> [_ w608]
            tunnel: ["" w605] -> w594
            frame False {
            }
            frame True {
              n252 = call "ASYNC_Adam_server.vi"("Values"=w609, "Channel Names"=w608) -> ("Scan Comments"=w606:string[])  [unwired: 1 in, 2 out]
              n253 = Index Array(array=w606, index=0) -> (element=w605:string)
            }
          }
        }
      }
      frame #18 {
        # "To automatically control the request for the University Stall chiller to run."
        n254 = while {
          tunnel: w614 -> [w622]
          tunnel: w613 -> [w623]
          shift-right: [w617] -> _
          shift-left: _ -> [w632]
          shift-left: _ -> [w631]
          shift-left: _ -> [w630]
          tunnel: [w616] -> w612
          tunnel: [w615] -> w611
          stop <- FALSE continue-if-true
          n255 = Build Array("EnFlo_Tunnel:Chiller_Pump:Enable" ("Desired Ch to Read"), "Aero_Tunnel:Cooling_Pump:Enable" ("Desired Ch to Read")) -> (w624:string[])
          n256 = call "Read_Earlier_Channels.vi"("Present scan array"=w622, "Ch names"=w623, "Desired Channels"=w624) -> ("Scan comments"=w615:string, "Index 0"=w621:dbl, "Index 1"=w620:dbl)  [unwired: 3 out]
          n257 = Build Array(w621, w620) -> (w619:dbl[])
          n258 = Greater?(x=w619, y=0.5) -> (0:w618:bool[])
          n259 = Or Array Elements(Boolean array=w618) -> (logical OR=w617:bool)
          n260 = Compound Arithmetic op=AND(w617, w632, invert w631, invert w630) -> (w628:bool)
          n261 = Compound Arithmetic op=AND(invert w617, invert w632, w631, w630) -> (w629:bool)
          n262 = Or(x=w628, y=w629) -> (x .or. y?=w627:bool)
          n263 = case shown="True" w627 {
            tunnel: w617 -> [_ w641]
            tunnel: [string[] [] ("Scan Comments") w636] -> w616
            frame False {
            }
            frame True {
              n264 = case shown="False" w641 {
                tunnel: [string[] ["University:Chilled Water:Requested"] ("Channel Names") string[] ["University:Chilled Water:Requested"] ("Channel Names")] -> w640
                tunnel: [1.0 ("y") 0.0 ("y")] -> w637
                frame True {
                }
                frame False {
                }
              }
              n265 = Array Size(array=w640) -> (size(s)=w638:i32)
              n266 = Initialize Array(w637, w638) -> (w639:dbl[])
              n267 = call "ASYNC_Adam_server.vi"("Values"=w639, "Channel Names"=w640) -> ("Scan Comments"=w636:string[])  [unwired: 1 in, 2 out]
            }
          }
        }
        n268 = Concatenate Strings(w612, w611) -> (w610:string)
      }
      frame #19 {
        # "Exercise the floor cooling valve once a week"
        n269 = while {
          shift-right: [w650] -> _
          shift-left: _ -> [w655]
          tunnel: w648 -> [w650]
          tunnel: w647 -> [w652]
          tunnel: [w649] -> w646
          stop <- TRUE stop-if-true
          n270 = Not Equal?(x=w650, y=w655) -> (x != y?=w653:bool)
          n271 = Compound Arithmetic op=AND(w653, w652) -> (w651:bool)
          n272 = case shown="True" w651 {
            tunnel: w650 -> [_ w662]
            tunnel: ["" w657] -> w649
            frame False {
            }
            frame True {
              n273 = Select(t=1.0, s=w662, f=0.0) -> (s? t:f=w663:dbl)
              n274 = Build Array(w663) -> (w666:dbl[])
              n275 = Build Array("EnFlo_Tunnel:Floor_Cooling:Enable") -> (w665:string[])
              n276 = call "ASYNC_Adam_server.vi"("Values"=w666, "Channel Names"=w665) -> ("Scan Comments"=w658:string[])  [unwired: 1 in, 2 out]
              n277 = Index Array(array=w658, index=0) -> (element=w657:string)
            }
          }
        }
      }
      frame #20 {
        n278 = Concatenate Strings(w672, w673, w674, w675, w676, w677, w678, w685, w684, w683, w682, w681, w680, w679, w670, w669, w668, w667) -> (→"Scan comment":string)
      }
    }
  }
